vi "Global Post Step Runtime Error ID.vi"() -> ()   [LabVIEW 2023, in "RFCalAndFixtureCharact.Common.lvlib"]
uses:
  RFCalAndFixtureCharact.Common.lvlib
panel:
  in  "PostStepRuntimeErrorCode":i32=-1
  in  "PostStepRuntimeError":string="PostStepRuntimeError"
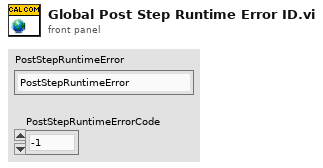
[diagram p1: front panel]
diagram:
